vi "log acq config errors.vi"(8 "error in (no error)":errorcluster, 11 "SPARC4_Channel in":refnum<class "SPARC4_Channel.lvclass">) -> (0 "error out":errorcluster, 3 "SPARC4_Channel out":refnum<class "SPARC4_Channel.lvclass">)   [LabVIEW 2018, in "SPARC4_Channel.lvclass"]
uses:
  SPARC4_Channel.lvclass
  C:/Users/Denis/Desktop/S4ACS/S4ACS/Channel/Channel.lvclass
  SPARC4_Channel.lvclass/SPARC4_Channel.ctl
  Channel/Channel.lvclass
panel:
  out "s4 acq config errors":T1
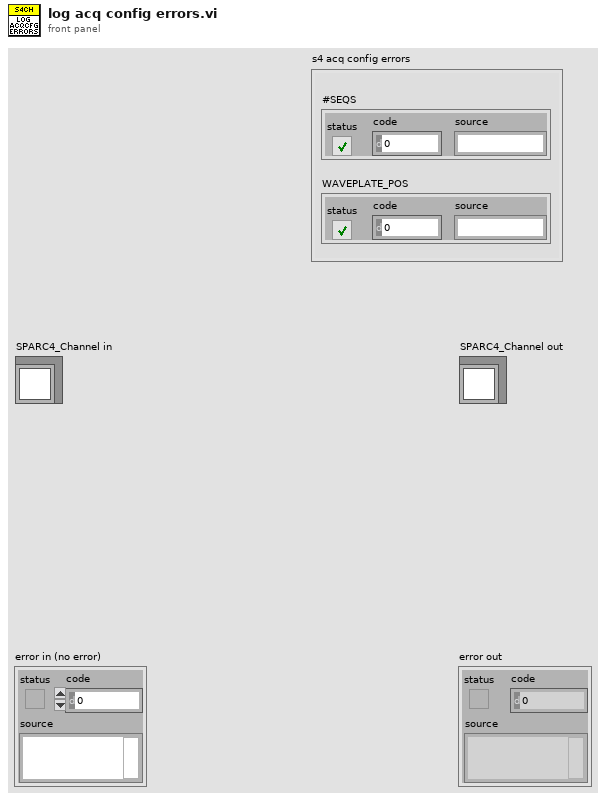
[diagram p1: front panel]
types:
  T1 = cluster{"#SEQS":errorcluster, "WAVEPLATE_POS":errorcluster}
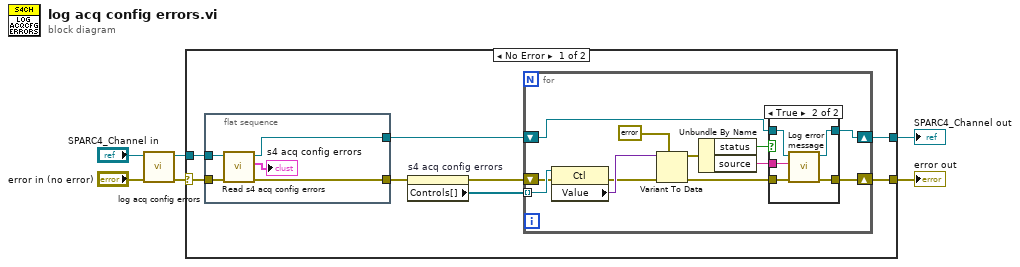
[diagram p0: block diagram]
diagram:
  n1 = call-parent "log acq config errors.vi"("error in (no error)"="error in (no error)", "Channel in"="SPARC4_Channel in") -> ("error out"=w4:errorcluster, "Channel out"=w2:refnum<class "SPARC4_Channel.lvclass">)  [unwired: 8 in]
  n2 = case shown="No Error" w4 {
    selector: w4 -> [w13 w40]
    tunnel: [w12 w40] -> w3
    tunnel: w2 -> [w14 w39]
    tunnel: [w11 w39] -> w1
    frame No Error {
      n3 = flat-sequence {
        tunnel: w14 -> [w19]
        tunnel: w13 -> [w18]
        tunnel: [w17] -> w9
        tunnel: [w16] -> w10
        frame #0 {
          n4 = call "Read s4 acq config errors.vi"("error in (no error)"=w18, "SPARC4_Channel in"=w19) -> ("error out"=w17:errorcluster, "s4 acq config errors"=→"s4 acq config errors":T1, "SPARC4_Channel out"=w16:refnum<class "SPARC4_Channel.lvclass">)  [unwired: 6 in, 1 out]
        }
      }
      n5 = property on="s4 acq config errors" class="Clust (strict)"(error in=w9) -> (error out=w8:errorcluster, "Controls[]"=w7:refnum<vi>[])  [unwired: 1 in, 1 out]
      n6 = for {
        shift-right: [w30] -> w11
        shift-left: w10 -> [w31]
        shift-right: [w29] -> w12
        shift-left: w8 -> [w26]
        tunnel: w7 -> [w28] mode=indexing
        n7 = property class="Ctl"(reference=w28, error in=w26) -> (error out=w25:errorcluster, "Value"=w27:variant)  [unwired: 1 out]
        n8 = Variant To Data(error in=w25, type=errorcluster {"status"=FALSE, "code"=0, "source"=""} ("error constant"), Variant=w27) -> (data=w22:errorcluster, error out=w23:errorcluster)
        n9 = Unbundle By Name(w22) -> ("status"=w20:bool, "source"=w21:string)
        n10 = case shown="True" w20 {
          tunnel: w31 -> [w33 w38]
          tunnel: [w33 w37] -> w30
          tunnel: [w32 w36] -> w29
          tunnel: w23 -> [w32 w35]
          tunnel: w21 -> [_ w34]
          frame False {
          }
          frame True {
            n11 = call "Log error message.vi"("error in (no error)"=w35, "String"=w34, "Channel in"=w38) -> ("error out"=w36:errorcluster, "Channel out"=w37:refnum<class "SPARC4_Channel.lvclass">)  [unwired: 7 in]
          }
        }
      }
    }
    frame Error {
    }
  }
  "error out" <- w3
  "SPARC4_Channel out" <- w1
